vi "Select Side Randomly.vi"(11 "Do not include this side":T1) -> (2 "Counter Side":T1, 3 "Side":T1)   [LabVIEW 2019, in "Day 15.lvlib"]
uses:
  Day 15.lvlib
  Day 11/Controls/Side.ctl
  <vilib>/numeric/Random Number (Range) I64.vi
  <vilib>/numeric/sub_Random U32.vi
  Day 11/Day 11.lvlib
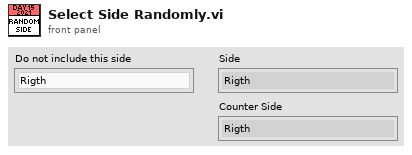
[diagram p1: front panel]
types:
  T1 = typedef "Day 11.lvlib/Side.ctl" = enum16{"Rigth", "Left", "Down", "Up", "Rigth Up", "Rigth Down", "Left Up", "Left Down"}
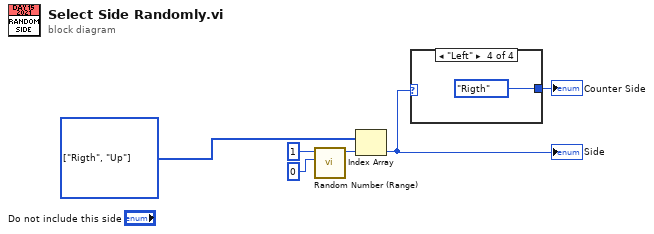
[diagram p0: block diagram]
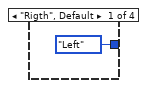
[diagram p2: hidden frame]
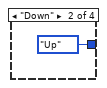
[diagram p3: hidden frame]
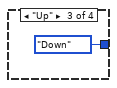
[diagram p4: hidden frame]
diagram:
  w1 = T1[] [enum."Rigth", enum."Up"] items=["Rigth", "Left", "Down", "Up", "Rigth Up", "Rigth Down", "Left Up", "Left Down"]
  n1 = call-poly <vilib>:"Random Number (Range).vi"("lower bound (-100)"=i64 0, "upper bound (100)"=i64 1) -> ("number"=w6:i64)  [unwired: 9 in]
  n2 = Index Array(array=w1, index=w6) -> (element=w3:T1)
  "Side" <- w3
  n3 = case shown="\"Left\"" w3 {
    tunnel: [Side."Left" ("Side") Side."Up" ("Side") Side."Down" ("Side") Side."Rigth" ("Side")] -> w2
    frame "Rigth", Default {
    }
    frame "Down" {
    }
    frame "Up" {
    }
    frame "Left" {
    }
  }
  "Counter Side" <- w2
